vi "sqltest.vi"   [LabVIEW 2024]
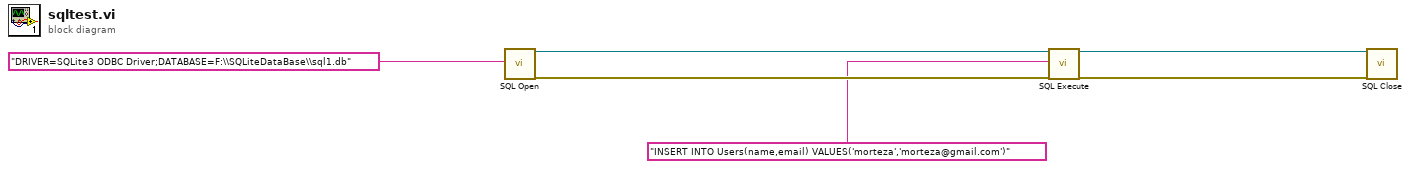
[diagram p0: block diagram]
diagram:
  n1 = call <vilib>:"SQL Open.vi"("ConnectionString In"="DRIVER=SQLite3 ODBC Driver;DATABASE=F:\\SQLiteDataBase\\sql1.db") -> ("Connection Out"=w5:refnum<k7>, "Error out"=w3:errorcluster)  [unwired: 17 in]
  n2 = call <vilib>:"SQL Execute.vi"("Connection In"=w5, "SQL Query"="INSERT INTO Users(name,email) VALUES('morteza','morteza@gmail.com')", "Error in (no error)"=w3) -> ("Connection Out"=w4:refnum<k7>, "Error out"=w2:errorcluster)  [unwired: 15 in]
  n3 = call <vilib>:"SQL Close.vi"("Connection In"=w4, "Error in (no error)"=w2) -> ()  [unwired: 17 in, 1 out]
